vi "Write Bounds.vi"(8 "error in (no error)":errorcluster, 10 "Rectangle":T1, 11 "Panel Object in":refnum<class "Panel Object.lvclass">) -> (0 "error out":errorcluster, 3 "Panel Object out":refnum<class "Panel Object.lvclass">)   [LabVIEW 2015, in "Panel Object.lvclass"]
uses:
  Panel Object.lvclass
  Typedefs/Rectangle--Cluster.ctl
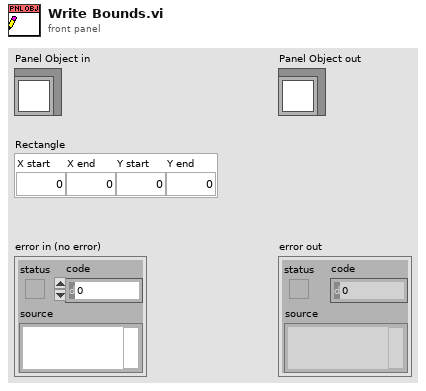
[diagram p1: front panel]
types:
  T1 = typedef "Rectangle--Cluster.ctl" = cluster{"X start":i32, "X end":i32, "Y start":i32, "Y end":i32}
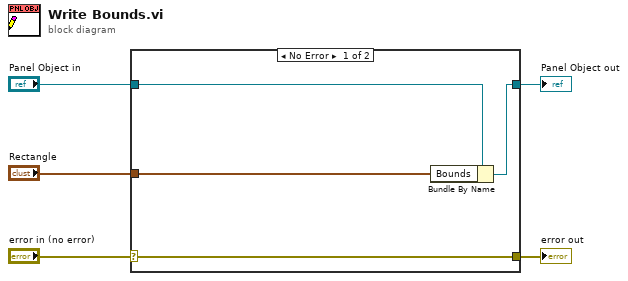
[diagram p0: block diagram]
diagram:
  n1 = case shown="No Error" "error in (no error)" {
    selector: "error in (no error)" -> [w9 w10]
    tunnel: [w9 w10] -> w4
    tunnel: [w7 w11] -> w2
    tunnel: "Panel Object in" -> [w8 w11]
    tunnel: "Rectangle" -> [w6 _]
    frame No Error {
      n2 = Bundle By Name(cluster=w8, "Bounds"=w6) -> (w7:refnum<class "Panel Object.lvclass">)
    }
    frame Error {
    }
  }
  "error out" <- w4
  "Panel Object out" <- w2
